vi "Test Fake DAQ.vi"() -> ()   [LabVIEW 2009]
uses:
  lib/DAQ IO/Daq Actions.ctl
  OperationManagerGlobal.vi
  lib/Data Access Objects/Metadata/LBCB Number.ctl
panel:
  out "L2 Servo Error":cluster{dbl[], "L1 LVDT & LC":dbl[]}[](graph)
  out "L2 LC":cluster{dbl[], "L1 LVDT & LC":dbl[]}[](graph)
  out "L2 LVDT":cluster{dbl[], "L1 LVDT & LC":dbl[]}[](graph)
  out "L1 Servo Error":cluster{dbl[], "L1 LVDT & LC":dbl[]}[](graph)
  out "L1 LC":cluster{dbl[], "L1 LVDT & LC":dbl[]}[](graph)
  in  "Plot Labels":string[](array[string])=["X1", "X2", "Y1", "Z1", "Z2", "Z3"]
  out "L1 LVDT":cluster{dbl[], "L1 LVDT & LC":dbl[]}[](graph)
  in  "LBCB Number":T1
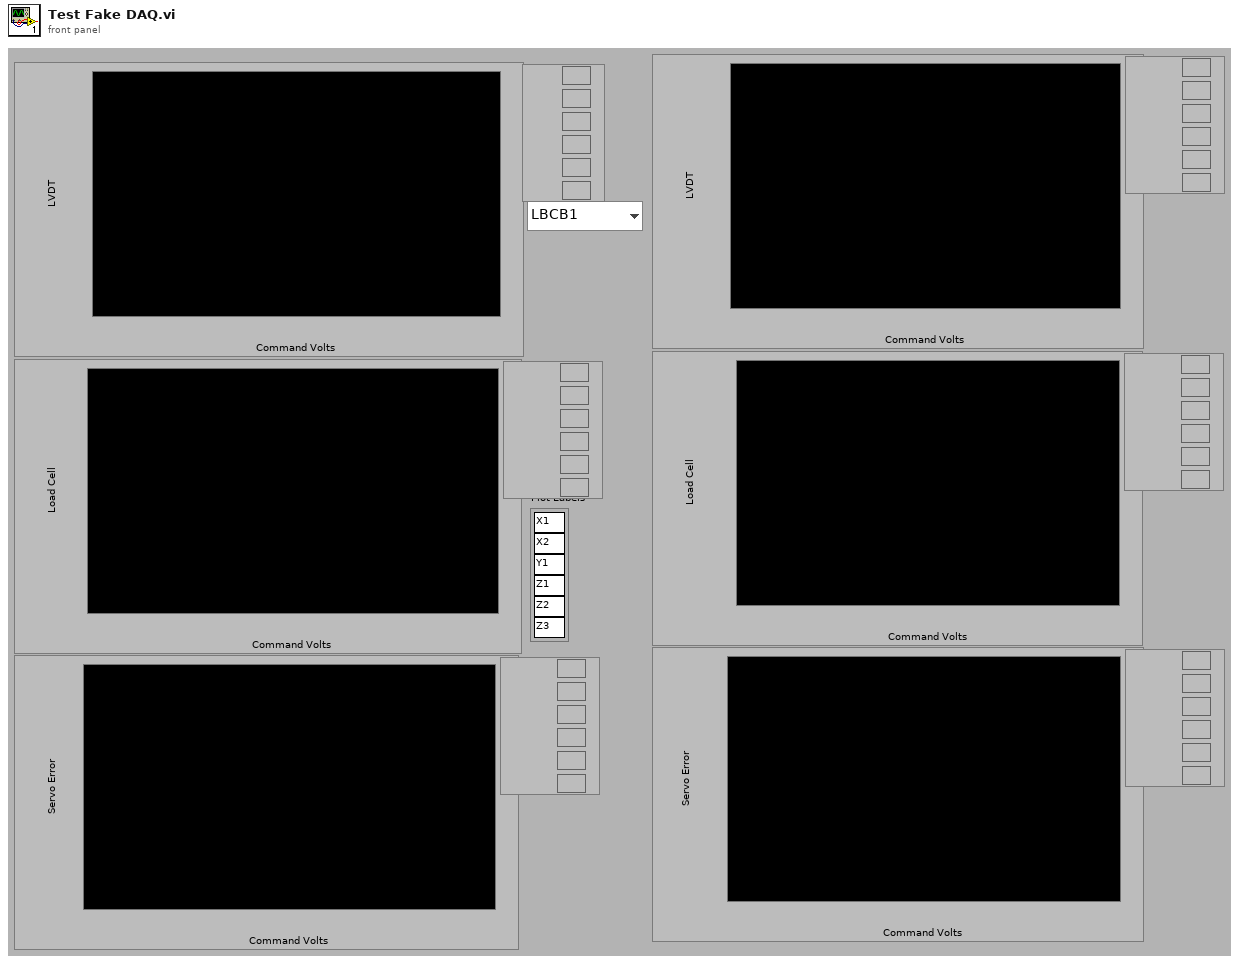
[diagram p1: front panel]
types:
  T1 = typedef "LBCB Number.ctl" = enum16{"LBCB1", "LBCB2"}
  T2 = typedef "Daq Actions.ctl" = enum16{"Init", "Send Commands", "Get Responses", "Stop"}
  T3 = cluster{"Command Sensitivities":dbl[], "Measured Sensitivities ":dbl[], "Absolute Offsets":dbl[], "Actuator Control Channels":refnum<k21>, "Actuator Measurement Channels":refnum<k21>, "Actuator Errors":dbl[], "Servo Error Channels":refnum<k21>, "Target Servo Errors":dbl[], "Control Setting":cluster{"Size":u16, "Type":u16, "Motion Center":dbl[], "Transformation Matrix":dbl[][]}, "Calib_C3":dbl[], "Calib_C2":dbl[], "Calib_C1":dbl[], "Calib_C0":dbl[], "LVDT_C3":dbl[], "LVDT_C2":dbl[], "LVDT_C1":dbl[], "LVDT_C0":dbl[], "Use\nPolynomial":bool}
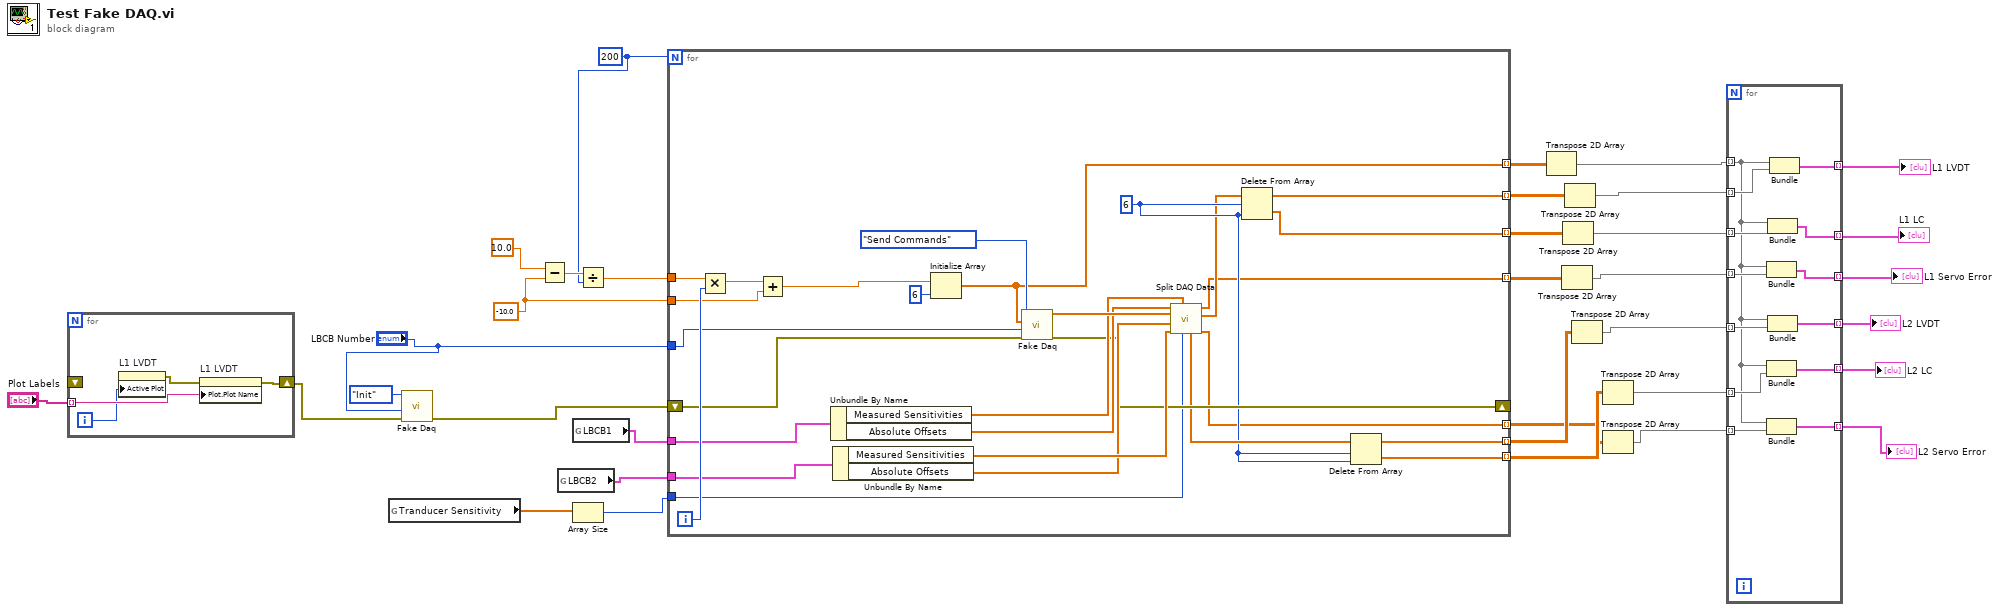
[diagram p0: block diagram]
diagram:
  w16 = -10.0
  w32 = 200
  n1 = for {
    tunnel: "Plot Labels" -> [w36] mode=indexing
    shift-right: [w37] -> w22
    shift-left: _ -> [_]
    i -> [w35]
    n2 = property on="L1 LVDT" class="XYGraph (strict)"("Active Plot"=w35) -> (error out=w38:errorcluster)  [unwired: 2 in, 1 out]
    n3 = property on="L1 LVDT" class="XYGraph (strict)"(error in=w38, "Plot.Plot Name"=w36) -> (error out=w37:errorcluster)  [unwired: 1 in, 1 out]
  }
  n4 = global read "OperationManagerGlobal.vi" "Tranducer Sensitivity"() -> (w26:dbl[])
  n5 = call "Fake Daq.vi"("error in (no error)"=w22, "LBCB Number"="LBCB Number", "Fake Daq Actions"=Daq_Actions."Init") -> ("error out"=w29:errorcluster)  [unwired: 1 in, 7 out]
  n6 = Subtract(x=10.0, y=w16) -> (x-y=w33:dbl)
  n7 = global read "OperationManagerGlobal.vi" "LBCB2"() -> (w27:T3)
  n8 = global read "OperationManagerGlobal.vi" "LBCB1"() -> (w28:T3)
  n9 = Array Size(array=w26) -> (size(s)=w25:i32)
  n10 = Divide(x=w33, y=w32) -> (x/y=w31:dbl)
  n11 = for {
    N: w32 -> [_]
    tunnel: w31 -> [w65]
    tunnel: "LBCB Number" -> [w60]
    shift-right: [w54] -> _
    shift-left: w29 -> [w59]
    tunnel: w28 -> [w50]
    tunnel: w27 -> [w49]
    tunnel: w25 -> [w48]
    tunnel: [w47] -> w21 mode=indexing
    tunnel: [w46] -> w20 mode=indexing
    tunnel: w16 -> [w44]
    tunnel: [w43] -> w15 mode=indexing
    tunnel: [w42] -> w12 mode=indexing
    tunnel: [w41] -> w9 mode=indexing
    tunnel: [w40] -> w8 mode=indexing
    tunnel: [w39] -> w7 mode=indexing
    i -> [w64]
    w52 = 6 ("length")
    n12 = Multiply(x=w65, y=w64) -> (x*y=w63:dbl)
    n13 = Add(x=w63, y=w44) -> (x+y=w45:dbl)
    n14 = Unbundle By Name(w50) -> ("Measured Sensitivities"=w58:dbl[], "Absolute Offsets"=w57:dbl[])
    n15 = Unbundle By Name(w49) -> ("Measured Sensitivities"=w56:dbl[], "Absolute Offsets"=w55:dbl[])
    n16 = Initialize Array(w45, 6 ("dimension size")) -> (w47:dbl[])
    n17 = call "Fake Daq.vi"("error in (no error)"=w59, "LBCB Number"=w60, "Commands"=w47, "Fake Daq Actions"=Daq_Actions."Send Commands") -> ("error out"=w54:errorcluster, "Responses"=w66:dbl[])  [unwired: 6 out]
    n18 = call "Split DAQ Data.vi"("Number of \nExternal \nChannels"=w48, "L1 Measured Sensitivities"=w58, "L2 Measured Sensitivities"=w56, "L2 Absolute Offsets"=w55, "Responses"=w66, "L1 Absolute Offsets"=w57) -> ("L2 Servo Error"=w39:dbl[], "L1 LVDT & LC"=w51:dbl[], "L1 Servo Error"=w42:dbl[], "L2 LVDT & LC"=w53:dbl[])  [unwired: 1 out]
    n19 = Delete From Array(array=w51, length=w52, index=w52) -> (deleted portion=w43:dbl[], array with subset deleted=w46:dbl[])
    n20 = Delete From Array(array=w53, length=w52, index=w52) -> (deleted portion=w40:dbl[], array with subset deleted=w41:dbl[])
  }
  n21 = Transpose 2D Array(2D array=w21) -> (transposed array=w18:dbl[][])
  n22 = Transpose 2D Array(2D array=w12) -> (transposed array=w11:dbl[][])
  n23 = Transpose 2D Array(2D array=w15) -> (transposed array=w14:dbl[][])
  n24 = Transpose 2D Array(2D array=w20) -> (transposed array=w17:dbl[][])
  n25 = Transpose 2D Array(2D array=w9) -> (transposed array=w6:dbl[][])
  n26 = Transpose 2D Array(2D array=w8) -> (transposed array=w5:dbl[][])
  n27 = Transpose 2D Array(2D array=w7) -> (transposed array=w4:dbl[][])
  n28 = for {
    tunnel: w18 -> [w70] mode=indexing
    tunnel: w17 -> [w79] mode=indexing
    tunnel: [w78] -> w19 mode=indexing
    tunnel: w14 -> [w77] mode=indexing
    tunnel: [w76] -> w13 mode=indexing
    tunnel: w11 -> [w75] mode=indexing
    tunnel: [w74] -> w10 mode=indexing
    tunnel: w6 -> [w73] mode=indexing
    tunnel: w5 -> [w72] mode=indexing
    tunnel: w4 -> [w71] mode=indexing
    tunnel: [w69] -> w3 mode=indexing
    tunnel: [w68] -> w2 mode=indexing
    tunnel: [w67] -> w1 mode=indexing
    n29 = Bundle(w70, w75) -> (w74:cluster{dbl[], dbl[]})  [unwired: 1 out]
    n30 = Bundle(w70, w72) -> (w68:cluster{dbl[], dbl[]})  [unwired: 1 out]
    n31 = Bundle(w70, w71) -> (w67:cluster{dbl[], dbl[]})  [unwired: 1 out]
    n32 = Bundle(w70, w77) -> (w76:cluster{dbl[], dbl[]})  [unwired: 1 out]
    n33 = Bundle(w70, w73) -> (w69:cluster{dbl[], dbl[]})  [unwired: 1 out]
    n34 = Bundle(w70, w79) -> (w78:cluster{dbl[], dbl[]})  [unwired: 1 out]
  }
  "L1 LVDT" <- w19
  "L1 LC" <- w13
  "L1 Servo Error" <- w10
  "L2 LVDT" <- w3
  "L2 LC" <- w2
  "L2 Servo Error" <- w1
